vi "damped sinusoid fit.vi"(7 "fitting parameters":T1 {"decay rate (1/sec)" scale=0.0..20000.0; "start phase (deg)" scale=-180.0..180.0; "frequency (Hz)" scale=0.0..20000.0; "amplitude (V)" scale=0.0..10.0}, 11 "time array in (s)":dbl[](array[numeric])) -> (0 "parameters array out":dbl[](array[numeric]), 2 "voltage array out (V)":dbl[](array[numeric]), 3 "time array out (s)":dbl[](array[numeric]))   [LabVIEW 2014]
uses:
  typedefs/damped wave parameter cluster.ctl
panel:
  # "see diagram"
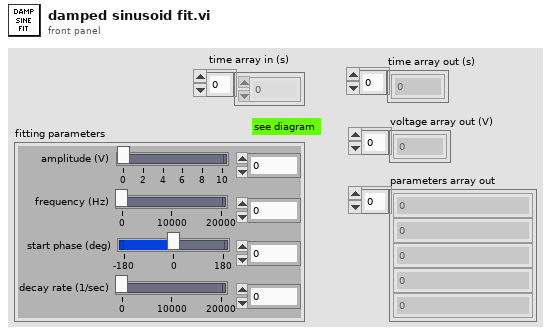
[diagram p1: front panel]
types:
  T1 = typedef "damped wave parameter cluster.ctl" = cluster{"amplitude (V)":dbl, "frequency (Hz)":dbl, "start phase (deg)":dbl, "decay rate (1/sec)":dbl}
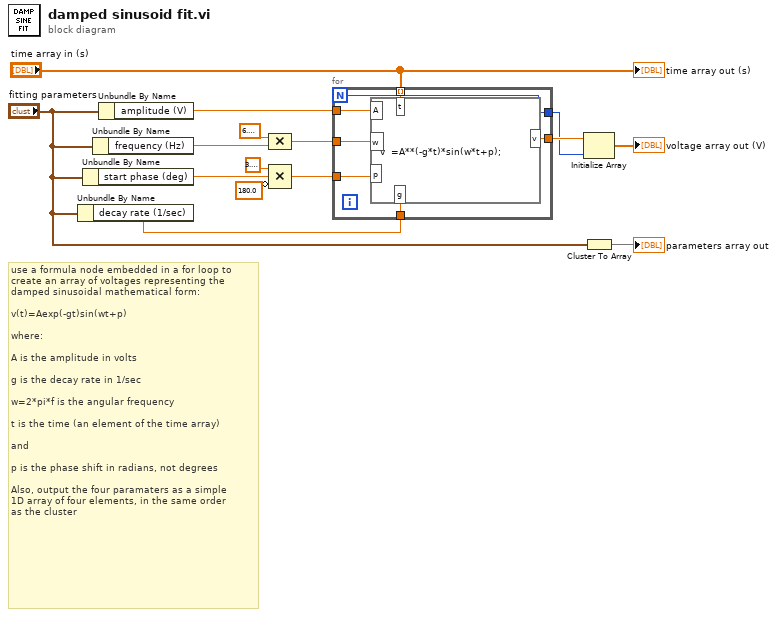
[diagram p0: block diagram]
diagram:
  # "use a formula node embedded in a for loop to \ncreate an array of voltages representing the \ndamped sinusoidal mathematical form:\n\nv(t)=Aexp(-gt)sin(wt+p)\n\nwhere:\n\nA is the amplitude in volts\n\ng is the decay rate in 1/sec\n\nw=2*pi*f is the angular frequency\n\nt is the time (an element of the time array)\n\nand\n\np is the phase shift in radians, not degrees\n\nAlso, output the four paramaters as a simple \n1D array of four elements, in the same order\nas the cluster"
  n1 = Unbundle By Name("fitting parameters") -> ("decay rate (1/sec)"=w6:dbl)
  n2 = Unbundle By Name("fitting parameters") -> ("start phase (deg)"=w11:dbl)
  n3 = Unbundle By Name("fitting parameters") -> ("frequency (Hz)"=w12:dbl)
  n4 = Unbundle By Name("fitting parameters") -> ("amplitude (V)"=w10:dbl)
  n5 = Compound Arithmetic op=MULTIPLY(6.283185307179586, w12) -> (w7:dbl)
  n6 = Compound Arithmetic op=MULTIPLY(3.141592653589793, w11, invert 180.0 ("value")) -> (w8:dbl)
  n7 = for {
    N -> [w16]
    tunnel: w10 -> [w22]
    tunnel: "time array in (s)" -> [w21] mode=indexing
    tunnel: w8 -> [w20]
    tunnel: w7 -> [w19]
    tunnel: w6 -> [w18]
    tunnel: [w17] -> w5
    tunnel: [w16] -> w4
    n8 = formula code="v  =A**(-g*t)*sin(w*t+p);"("A"=w22, "t"=w21, "w"=w19, "p"=w20, "g"=w18) -> ("v"=w17:dbl)
  }
  n9 = Initialize Array(w5, w4) -> (→"voltage array out (V)":dbl[])
  n10 = Cluster To Array(cluster="fitting parameters") -> (array=→"parameters array out":dbl[])
  "time array out (s)" <- "time array in (s)"
